vi "Utility_Merge ROIs.vi"(8 "error in (no error)":errorcluster, 11 "QSM_ShiftRegister_TEST in":T2 {"ROI Process"."Particle Variables" items=["Center of Mass X", "Center of Mass Y", "First Pixel X", "First Pixel Y", "Bounding Rect Left", "Bounding Rect Top", "Bounding Rect Right", "Bounding Rect Bottom", "Max Feret Diameter Start X", "Max Feret Diameter Start Y", "Max Feret Diameter End X", "Max Feret Diameter End Y", "Max Horiz. Segment Length Left", "Max Horiz. Segment Length Right", "Max Horiz. Segment Length Row", "-", "Bounding Rect Width", "Bounding Rect Height", "Bounding Rect Diagonal", "Perimeter", "Convex Hull Perimeter", "Holes' Perimeter", "Max Feret Diameter", "Equivalent Ellipse Major Axis", "Equivalent Ellipse Minor Axis", "Equivalent Ellipse Minor Axis (Feret)", "Equivalent Rect Long Side", "Equivalent Rect Short Side", "Equivalent Rect Diagonal", "Equivalent Rect Short Side (Feret)", "Average Horiz. Segment Length", "Average Vert. Segment Length", "Hydraulic Radius", "Waddel Disk Diameter", "-", "Area", "Holes' Area", "Particle & Holes' Area", "Convex Hull Area", "Image Area", "-", "Number of Holes", "Number of Horiz. Segments", "Number of Vert. Segments", "-", "Orientation", "Max Feret Diameter Orientation", "-", "% Area/Image Area", "% Area/(Particle & Holes' Area)", "Ratio of Equivalent Ellipse Axes", "Ratio of Equivalent Rect Sides", "-", "Elongation Factor", "Compactness Factor", "Heywood Circularity Factor", "Type Factor", "-", "Sum X", "Sum Y", "Sum XX", "Sum XY", "Sum YY", "Sum XXX", "Sum XXY", "Sum XYY", "Sum YYY", "-", "Moment of Inertia XX", "Moment of Inertia XY", "Moment of Inertia YY", "Moment of Inertia XXX", "Moment of Inertia XXY", "Moment of Inertia XYY", "Moment of Inertia YYY", "Norm. Moment of Inertia XX", "Norm. Moment of Inertia XY", "Norm. Moment of Inertia YY", "Norm. Moment of Inertia XXX", "Norm. Moment of Inertia XXY", "Norm. Moment of Inertia XYY", "Norm. Moment of Inertia YYY", "Hu Moment 1", "Hu Moment 2", "Hu Moment 3", "Hu Moment 4", "Hu Moment 5", "Hu Moment 6", "Hu Moment 7"]; "ROI Process"."Particle Measurements (Pixels)" format="%.2f"; "ROI Process"."ROIS"."Contours"."Type" items=["No Selection", "Point", "Line", "Rectangle", "Oval", "Polygon", "Freehand Region", "Annulus", "Unused2", "Unused3", "Broken Line", "Freehand Line", "Rotated Rectangle"]; "Single Image Results"."ROI Results"."LIMLOCALMETADATA"."dTimeMSec" format="%.2f"}) -> (0 "error out":errorcluster, 2 "ROI":T1 {"Contours"."Type" items=["No Selection", "Point", "Line", "Rectangle", "Oval", "Polygon", "Freehand Region", "Annulus", "Unused2", "Unused3", "Broken Line", "Freehand Line", "Rotated Rectangle"]})   [LabVIEW 2014]
uses:
  QSM/Queue_TEST/Controls/QSM_ShiftRegister.ctl
  QSM/QueueMaintenance/TypeDef/QSMRef_ALL.ctl
  QSM/Queue_TESTGUIUPDATE/Controls/QSM_Reference.ctl
  QSM/Queue_TESTGUIUPDATE/Controls/QSM_DataType.ctl
  QSM/Queue_TESTGUIUPDATE/Controls/QSM_RunStates.ctl
  QSM/Queue_TEST/Controls/QSM_Reference.ctl
  QSM/Queue_TEST/Controls/QSM_DataType.ctl
  QSM/Queue_TEST/Controls/QSM_RunStates.ctl
  Custom Controls/cluster - Image Results.ctl
  ND2_Reader_32bit/controls/cluster_LIMLOCALMETADATA.ctl
  QSM/Queue_TESTGUIUPDATE/GUIUpdateQSM.lvlib
  QSM/Queue_TEST/TestQSM.lvlib
  QSM/QueueMaintenance/QueueMaintenance.lvlib
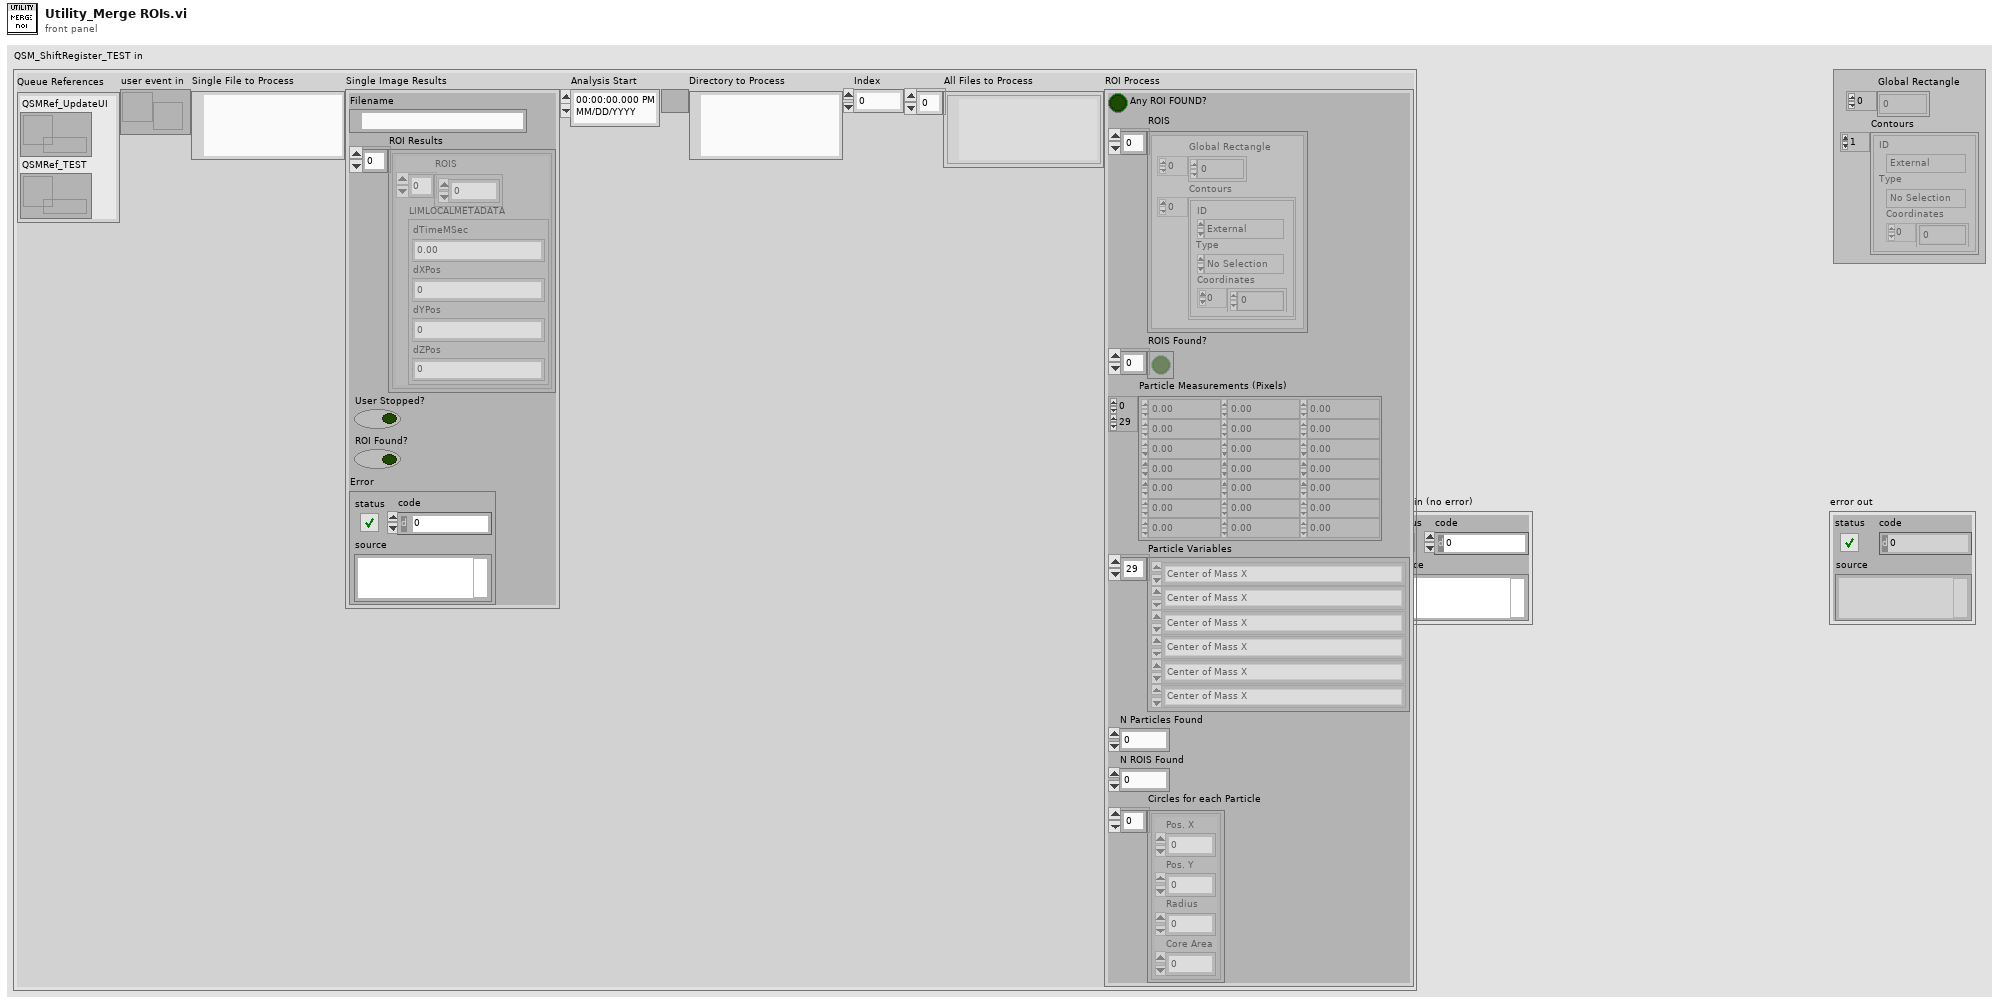
[diagram p1: front panel]
types:
  T1 = typedef "ROI Descriptor" = cluster{"Global Rectangle":i32[], "Contours":cluster{"ID":enum32{"External", "Internal"}, "Type":u32, "Coordinates":i32[]}[]}
  T2 = typedef "TestQSM.lvlib/QSM_ShiftRegister.ctl" = cluster{"Queue References":T3, "user event in":refnum<user-event>, "Single File to Process":path, "Single Image Results":T6, "Analysis Start":timestamp, "Directory to Process":path, "Index":i32, "All Files to Process":path[], "ROI Process":cluster{"Any ROI FOUND?":bool, "ROIS":T1[], "ROIS Found?":bool[], "Particle Measurements (Pixels)":dbl[][], "Particle Variables":i32[], "N Particles Found":i32, "N ROIS Found":i32, "Circles for each Particle":cluster{"Pos. X":i32, "Pos. Y":i32, "Radius":i32, "Core Area":i32}[]}}
  T3 = typedef "QueueMaintenance.lvlib/QSMRef_ALL.ctl" = cluster{"QSMRef_UpdateUI":T4, "QSMRef_TEST":T5}
  T4 = typedef "GUIUpdateQSM.lvlib/QSM_Reference.ctl" = refnum<queue>
  T5 = typedef "TestQSM.lvlib/QSM_Reference.ctl" = refnum<queue>
  T6 = typedef "cluster - Image Results.ctl" = cluster{"Filename":path, "ROI Results":cluster{"ROIS":dbl[], "LIMLOCALMETADATA":T7}[], "User Stopped?":bool, "ROI Found?":bool, "Error":errorcluster}
  T7 = typedef "cluster_LIMLOCALMETADATA.ctl" = cluster{"dTimeMSec":dbl, "dXPos":dbl, "dYPos":dbl, "dZPos":dbl}
  T8 = cluster{"ID":enum32{"External", "Internal"}, "Type":u32, "Coordinates":i32[]}[]
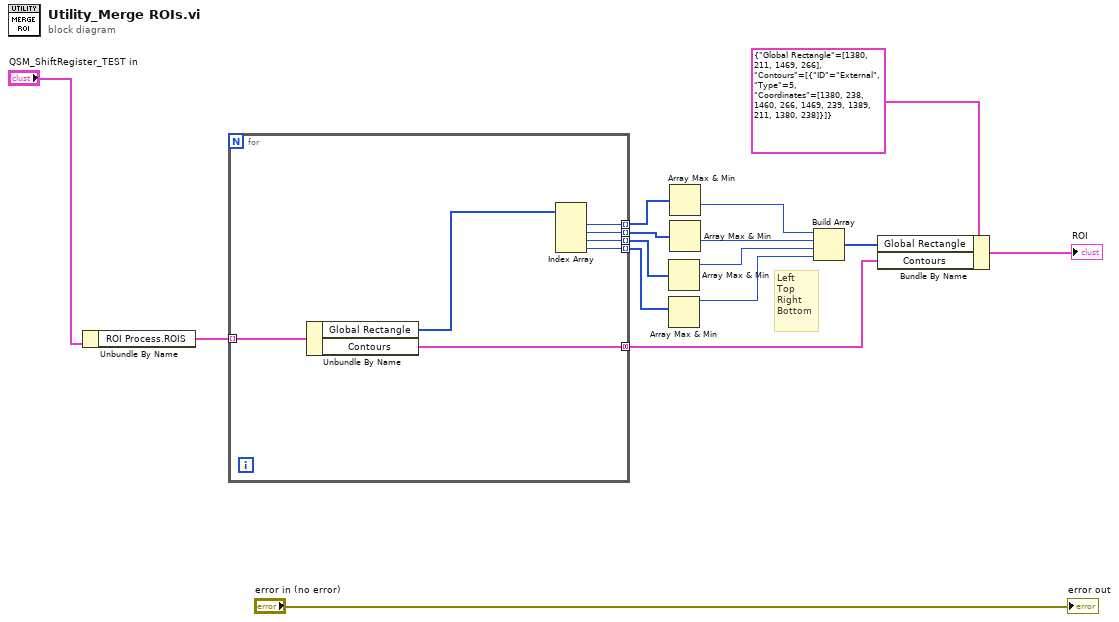
[diagram p0: block diagram]
diagram:
  # "Left\nTop\nRight\nBottom"
  n1 = Unbundle By Name("QSM_ShiftRegister_TEST in") -> ("ROI Process.ROIS"=w1:T1[])
  n2 = for {
    tunnel: w1 -> [w22] mode=indexing
    tunnel: [w21] -> w13 mode=concatenating
    tunnel: [w19] -> w11 mode=indexing
    tunnel: [w18] -> w10 mode=indexing
    tunnel: [w17] -> w9 mode=indexing
    tunnel: [w16] -> w8 mode=indexing
    n3 = Unbundle By Name(w22) -> ("Global Rectangle"=w20:i32[], "Contours"=w21:T8)
    n4 = Index Array(array=w20) -> (element #1=w19:i32, element #2=w18:i32, element #3=w17:i32, element #4=w16:i32)  [unwired: 4 in]
  }
  n5 = Array Max & Min(array=w9) -> (max value=w4:i32)  [unwired: 3 out]
  n6 = Array Max & Min(array=w8) -> (max value=w3:i32)  [unwired: 3 out]
  n7 = Array Max & Min(array=w11) -> (min value=w7:i32)  [unwired: 3 out]
  n8 = Array Max & Min(array=w10) -> (min value=w5:i32)  [unwired: 3 out]
  n9 = Build Array(w7, w5, w4, w3) -> (w6:i32[])
  n10 = Bundle By Name(cluster=T1 {"Global Rectangle"=[1380, 211, 1469, 266], "Contours"=[{"ID"=enum."External", "Type"=5, "Coordinates"=[1380, 238, 1460, 266, 1469, 239, 1389, 211, 1380, 238]}]} ("ROI"), "Global Rectangle"=w6, "Contours"=w13) -> (→"ROI":T1)
  "error out" <- "error in (no error)"
